vi "MarkerLeave.vi"(4 "User Parameter":variant, 5 "Event Data":cluster{"sender":refnum<k24>, "e":refnum<k24>}, 6 "Control Ref":refnum<k24>, 7 "Event Common Data":T1) -> ()   [LabVIEW 2014]
uses:
  C:/Robotic Systems/Products/AgFalcon/Software/Ground Station/Data/Mapping DLL/GMap.NET.WindowsForms.dll
  Data/Mapping DLL/GMap.NET.WindowsForms.dll
  Controls/GMap Mouse States.ctl
  FGVs/GMap Mouse State/Methods/SET Mouse State.vi
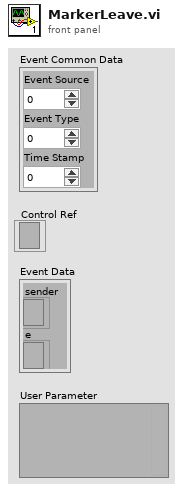
[diagram p1: front panel]
types:
  T1 = cluster{"Event Source":i32, "Event Type":u32, "Time Stamp":u32}
  T2 = typedef "GMap Mouse States.ctl" = enum16{"Mouse Down", "Mouse Up"}
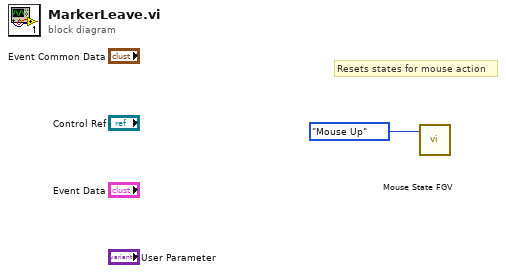
[diagram p0: block diagram]
diagram:
  # "Resets states for mouse action"
  n1 = call-poly "Mouse State FGV.vi"("Mouse State In"=GMap_Mouse_States."Mouse Up") -> ()  [unwired: 10 in, 1 out]
